vi "Manipulation3_2.vi"() -> ()   [LabVIEW 2017]
uses:
  Control 1.ctl
panel:
  out "Cluster 3":T1
  out "Cluster 4":T1
  out "Cluster 2":T1
  out "Cluster":T1
  in  "stop":bool
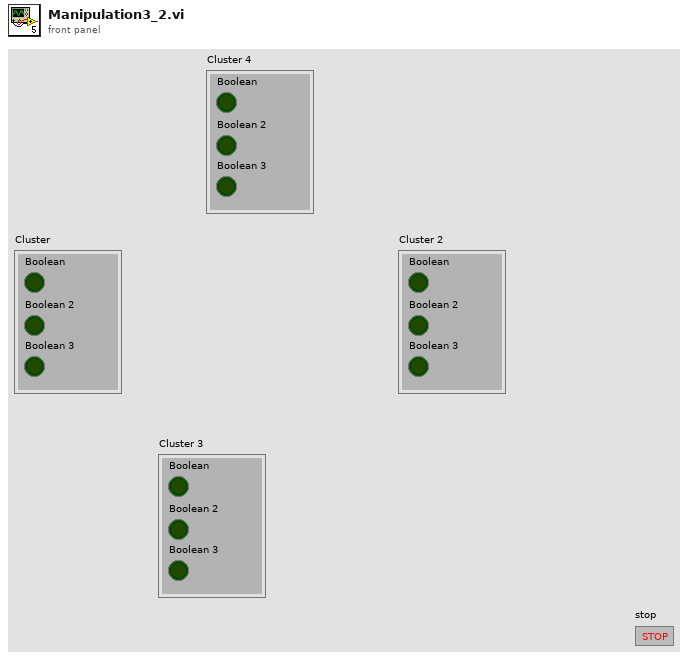
[diagram p1: front panel]
types:
  T1 = cluster{"Boolean":bool, "Boolean 2":bool, "Boolean 3":bool}
  T2 = typedef "Control 1.ctl" = enum16{"Vert", "Orange", "Rouge", "Rouge2"}
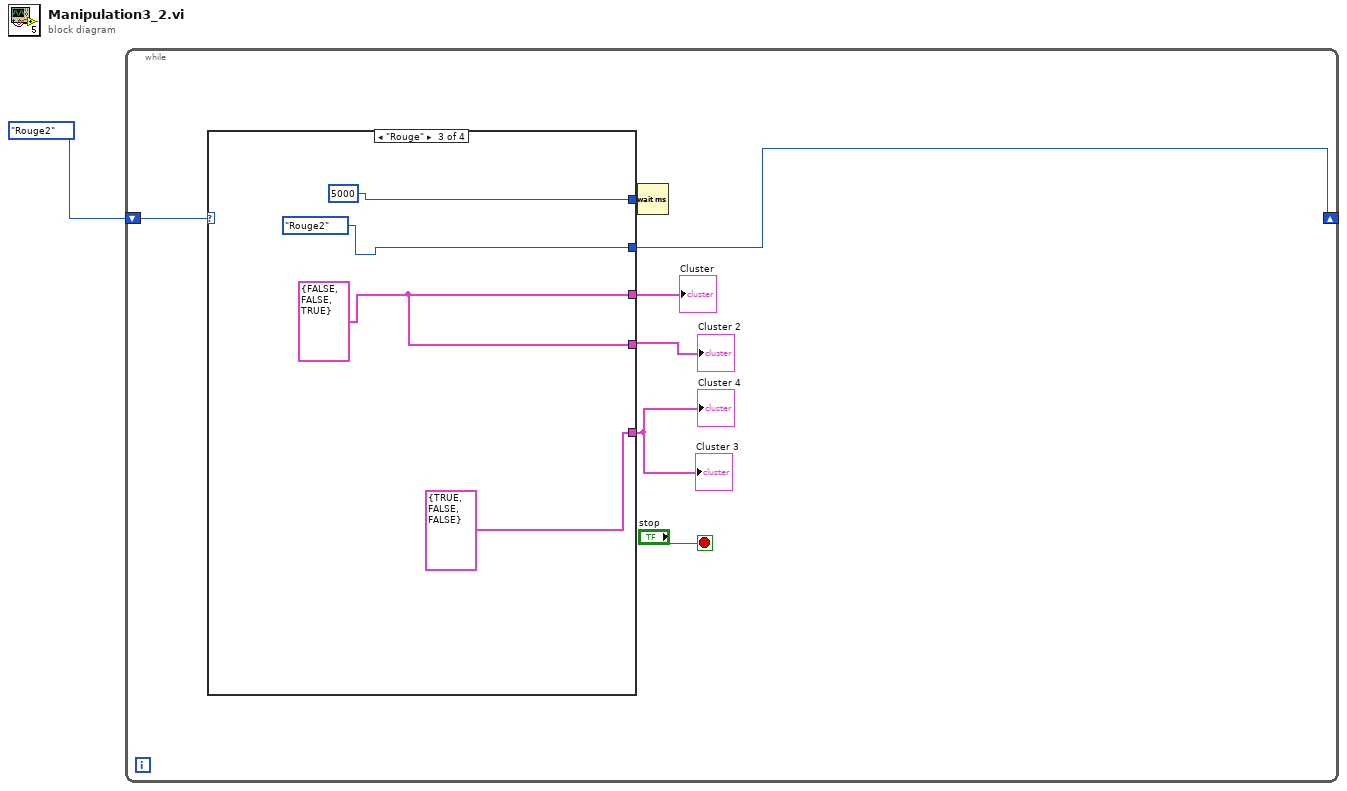
[diagram p0: block diagram]
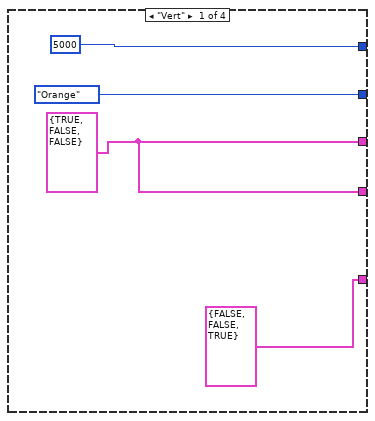
[diagram p2: hidden frame]
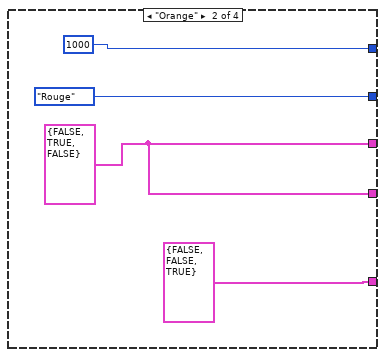
[diagram p3: hidden frame]
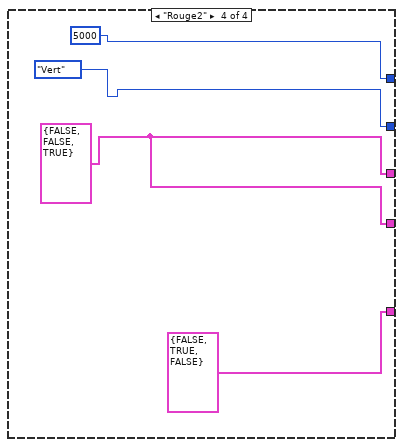
[diagram p4: hidden frame]
diagram:
  n1 = while {
    shift-right: [w4] -> _
    shift-left: Control_1."Rouge2" -> [w3]
    stop <- "stop" stop-if-true
    n2 = case shown="\"Rouge\"" w3 {
      tunnel: [5000 1000 5000 5000] -> w7
      tunnel: [enum16{"Vert", "Orange", "Rouge"}."Orange" enum16{"Vert", "Orange", "Rouge"}."Rouge" enum16{"Vert", "Orange", "Rouge", "Rouge2"}."Rouge2" ("Enum") enum16{"Vert", "Orange", "Rouge", "Rouge2"}."Vert" ("Enum")] -> w4
      tunnel: [w10 w14 w19 w23] -> w6
      tunnel: [w10 w14 w19 w23] -> w5
      tunnel: [cluster{bool, bool, bool} {FALSE, FALSE, TRUE} cluster{bool, bool, bool} {FALSE, FALSE, TRUE} cluster{bool, bool, bool} {TRUE, FALSE, FALSE} cluster{bool, bool, bool} {FALSE, TRUE, FALSE}] -> w2
      frame "Vert" {
        w10 = cluster{bool, bool, bool} {TRUE, FALSE, FALSE}
      }
      frame "Orange" {
        w14 = cluster{bool, bool, bool} {FALSE, TRUE, FALSE}
      }
      frame "Rouge" {
        w19 = cluster{bool, bool, bool} {FALSE, FALSE, TRUE}
      }
      frame "Rouge2" {
        w23 = cluster{bool, bool, bool} {FALSE, FALSE, TRUE}
      }
    }
    "Cluster" <- w6
    "Cluster 2" <- w5
    "Cluster 4" <- w2
    "Cluster 3" <- w2
    n3 = Wait (ms)(milliseconds to wait=w7) -> ()  [unwired: 1 out]
  }
